vi "Write OfficeTron3000.vi"(10 "OfficeTron3000":refnum<class "OfficeTron3000.lvclass">, 11 "OT3IPrinter In":refnum<class "OT3IPrinter.lvclass">) -> (3 "OT3IPrinter Out":refnum<class "OT3IPrinter.lvclass">)   [LabVIEW 2018, in "OfficeTron3000.lvlib" / "OT3IPrinter.lvclass"]
uses:
  OT3IPrinter.lvclass
  OfficeTron3000/OfficeTron3000.lvclass
  OT3IPrinter.lvclass/OT3IPrinter.ctl
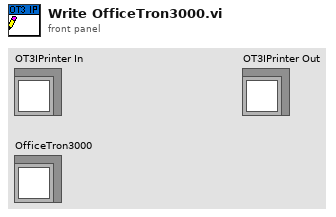
[diagram p1: front panel]
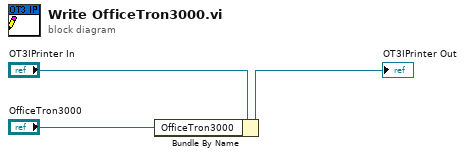
[diagram p0: block diagram]
diagram:
  n1 = Bundle By Name(cluster="OT3IPrinter In", "OfficeTron3000"="OfficeTron3000") -> (→"OT3IPrinter Out":refnum<class "OT3IPrinter.lvclass">)
